vi "outputs.vi"() -> ()   [LabVIEW 2020]
doc: "This global variable contains current robot state information and actuator setpoints."
panel:
  out "Piston_2_Command":bool
  out "Piston_1_Command":bool
  out "Piston_0_Command":bool
  out "Motor_15_Command":dbl
  out "Motor_14_Command":dbl
  out "Motor_13_Command":dbl
  out "Motor_12_Command":dbl
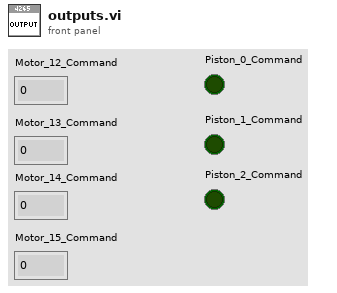
[diagram p1: front panel]
diagram:
